vi "Queue Is Nested.vi"(10 "Alias":string, 11 "Base Queue jettl in":refnum<class "Base Queue jettl.lvclass">) -> (2 "Queue Is Nested?":bool, 3 "Base Queue jettl out":refnum<class "Base Queue jettl.lvclass">)   [LabVIEW 2021, in "jettl.lvlib" / "Base Queue jettl.lvlib" / "Base Queue jettl.lvclass"]
uses:
  Base Queue jettl.lvclass
  C:/git/jettl/src/jettl/jettl/jettl.lvclass
  Base Queue jettl.lvclass/Base Queue jettl.ctl
  jettl.lvlib
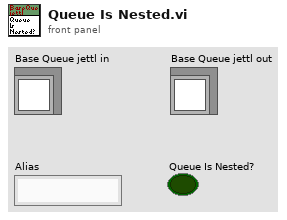
[diagram p1: front panel]
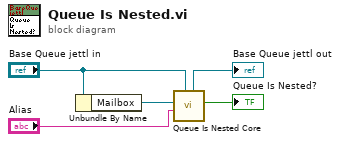
[diagram p0: block diagram]
diagram:
  n1 = Unbundle By Name("Base Queue jettl in") -> ("Mailbox"=w4:refnum<data-value>)
  n2 = call "Queue Is Nested Core.vi"("jettl in"="Base Queue jettl in", "Alias"="Alias", "Queue Mailbox"=w4) -> ("Queue Is Nested?"=→"Queue Is Nested?":bool, "jettl out"=→"Base Queue jettl out":refnum<class "Base Queue jettl.lvclass">)  [unwired: 7 in]
